vi "Get Leaf Notifier.vi"(8 "error in (no error)":errorcluster, 10 "ID In":i64[](array[numeric]), 11 "Root Actor in":refnum<class "Root Actor.lvclass">) -> (0 "error out":errorcluster, 2 "Node Notifier":T1, 3 "Root Actor out":refnum<class "Root Actor.lvclass">)   [LabVIEW 2019, in "Root Actor.lvclass"]
uses:
  Root Actor.lvclass
  System Actor/Type Def/Actor Notifier.ctl
  Root Actor.lvclass/Root Actor.ctl
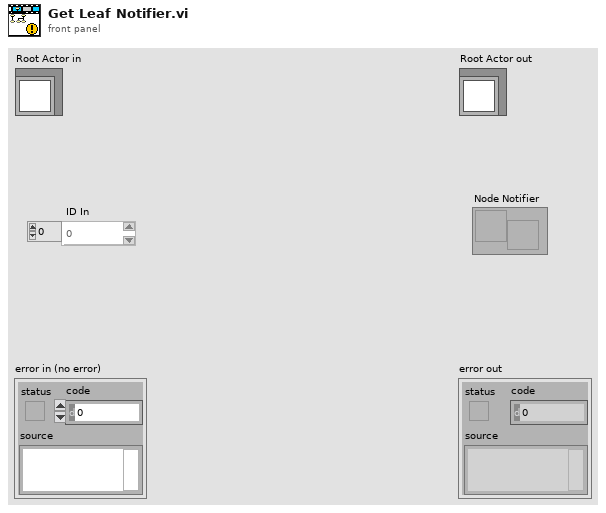
[diagram p1: front panel]
types:
  T1 = typedef "Actor Notifier.ctl" = refnum<notifier>
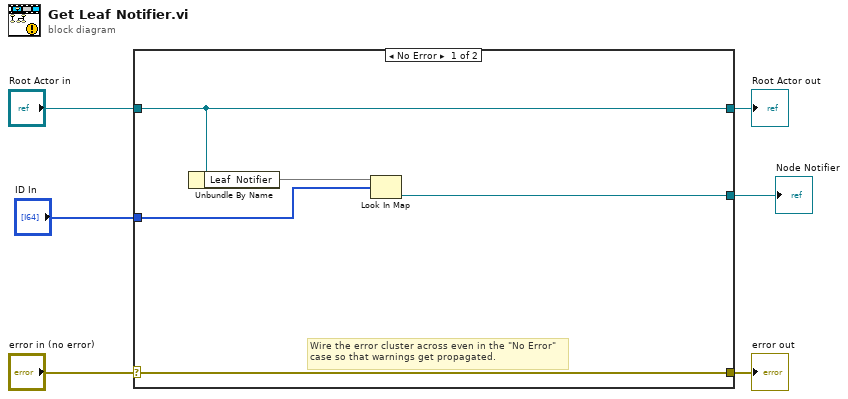
[diagram p0: block diagram]
diagram:
  n1 = case shown="No Error" "error in (no error)" {
    selector: "error in (no error)" -> [w11 w13]
    tunnel: [w11 w13] -> w5
    tunnel: [w10 w12] -> w3
    tunnel: "Root Actor in" -> [w10 w12]
    tunnel: "ID In" -> [w8 _]
    tunnel: [w7 _] -> w1
    frame No Error {
      # "Wire the error cluster across even in the \"No Error\"\ncase so that warnings get propagated."
      n2 = Unbundle By Name(w10) -> ("Leaf  Notifier"=w9:map{i64[], T1})
      n3 = Look In Map(map=w9, key=w8) -> (value=w7:T1)  [unwired: 1 in, 1 out]
    }
    frame Error {
    }
  }
  "error out" <- w5
  "Root Actor out" <- w3
  "Node Notifier" <- w1
